vi "polynom.vi"(3 "error in (no error)":errorcluster, 4 "value":dbl, 5 "array":dbl[][](array[numeric])) -> (0 "error out":errorcluster, 2 "result value":dbl)   [LabVIEW 2014, in "Array.lvlib"]
doc: "Return polynom from value. Every row in array contain A_i, B_i. The result will be summa(A_i*(x-B_i)^i)"
uses:
  Array.lvlib
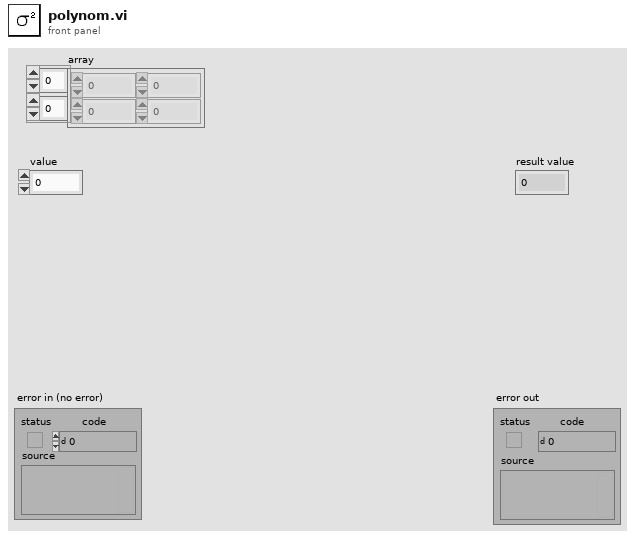
[diagram p1: front panel]
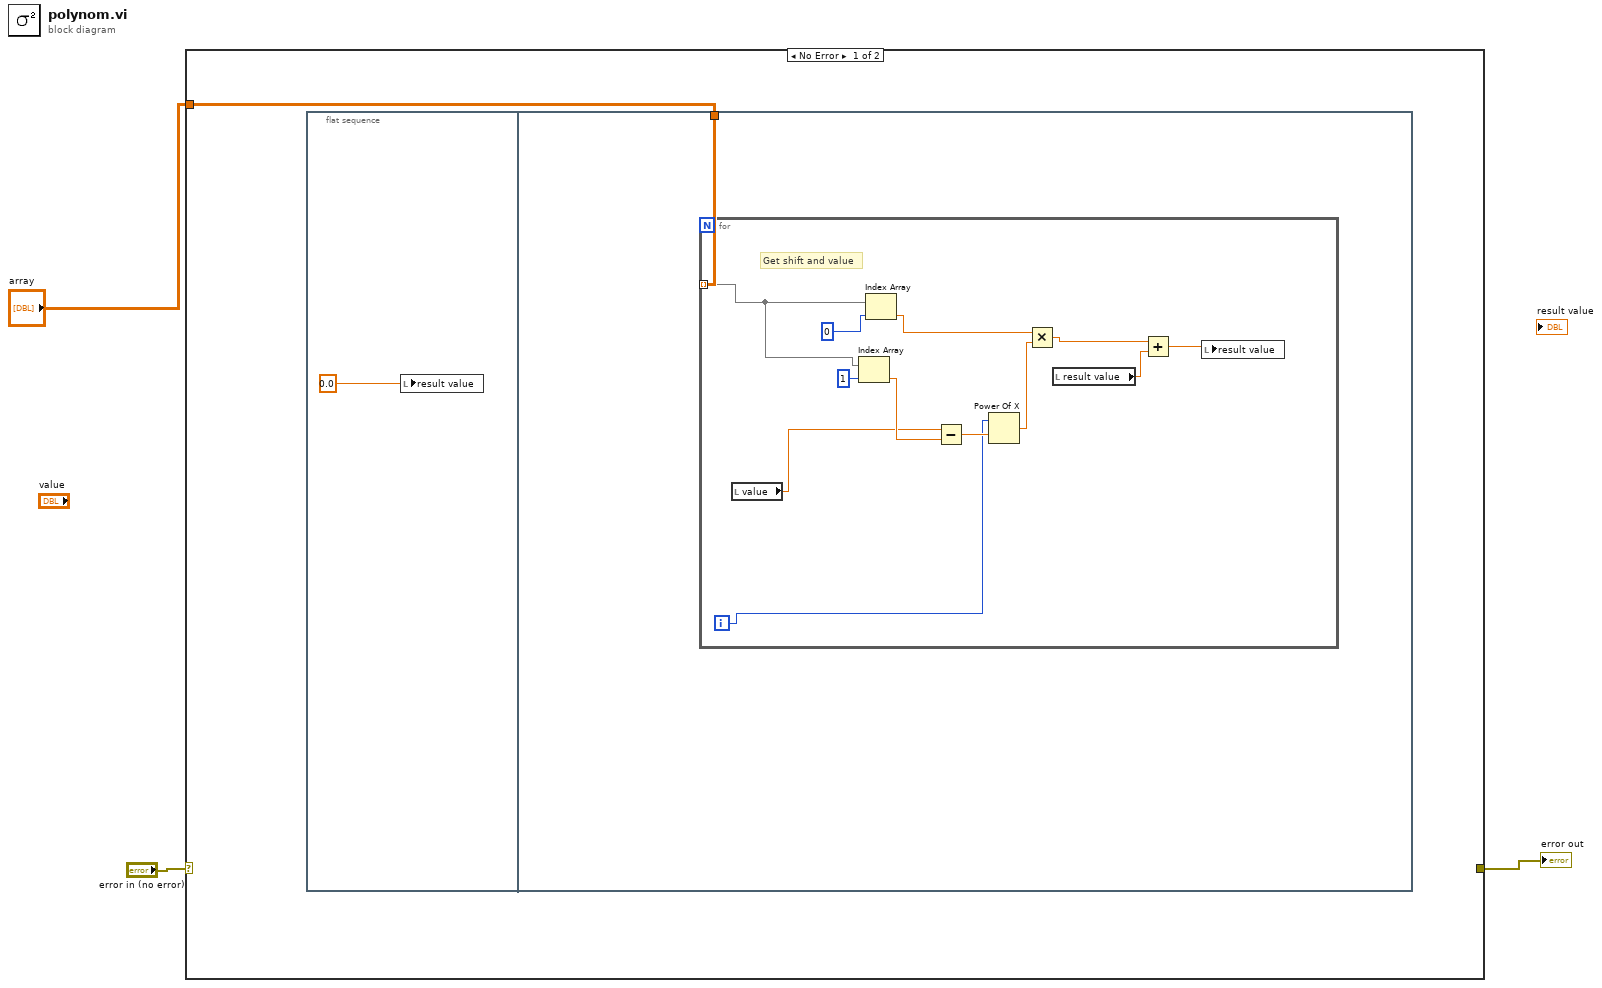
[diagram p0: block diagram]
diagram:
  n1 = case shown="No Error" "error in (no error)" {
    selector: "error in (no error)" -> [_ w19]
    tunnel: [_ w19] -> w2
    tunnel: "array" -> [w4 _]
    frame No Error {
      n2 = flat-sequence {
        tunnel: w4 -> [w6]
        frame #0 {
          n3 = local write "result value"(0.0) -> ()
        }
        frame #1 {
          n4 = for {
            tunnel: w6 -> [w16] mode=indexing
            i -> [w7]
            # "Get shift and value"
            n5 = local read "value"() -> (w14:dbl)
            n6 = Index Array(array=w16, index=1) -> (element=w15:dbl)
            n7 = Index Array(array=w16, index=0 ("index (dim 6)")) -> (element=w12:dbl)
            n8 = Subtract(x=w14, y=w15) -> (x-y=w13:dbl)
            n9 = Power Of X(1:w13, 2:w7) -> (0:w11:dbl)
            n10 = Multiply(x=w12, y=w11) -> (x*y=w10:dbl)
            n11 = local read "result value"() -> (w9:dbl)
            n12 = Add(x=w10, y=w9) -> (x+y=w8:dbl)
            n13 = local write "result value"(w8) -> ()
          }
        }
      }
    }
    frame Error {
    }
  }
  "error out" <- w2
